vi "Configure Trigger Source [TRG].vi"(8 "error in (no error)":errorcluster, 9 "trigger source (External)":i32(ring)=1 items=["Internal"=3, "External"=1, "Software Trigger Function"=2, "PXI TRIG0 or VXI TTL0"=111, "PXI TRIG1 or VXI TTL1"=112, "PXI TRIG2 or VXI TTL2"=113, "PXI TRIG3 or VXI TTL3"=114, "PXI TRIG4 or VXI TTL4"=115, "PXI TRIG5 or VXI TTL5"=116, "PXI TRIG6 or VXI TTL6"=117, "PXI TRIG7 or VXI TTL7"=118, "ECL0"=119, "ECL1"=120, "PXI Star"=131, "RTSI 0"=141, "RTSI 1"=142, "RTSI 2"=143, "RTSI 3"=144, "RTSI 4"=145, "RTSI 5"=146, "RTSI 6"=147], 10 "channel name (\"CHANNEL1\")":string="CHANNEL1", 11 "CS++Fgen in":refnum<class "CS++Fgen.lvclass">) -> (0 "error out":errorcluster, 3 "CS++Fgen out":refnum<class "CS++Fgen.lvclass">)   [LabVIEW 2013, in "CS++Fgen.lvlib" / "CS++Fgen.lvclass"]
doc: "This VI configures the trigger source for a channel.\n\nNotes:\n\n(1) This VI is part of the IviFgenTrigger [TRG] extension group."
uses:
  CS++Fgen.lvclass
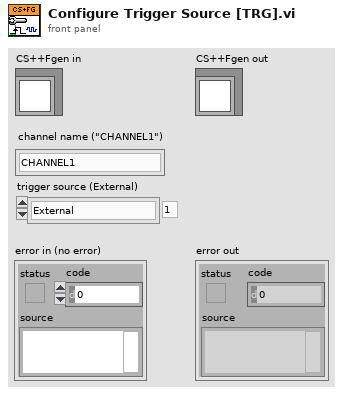
[diagram p1: front panel]
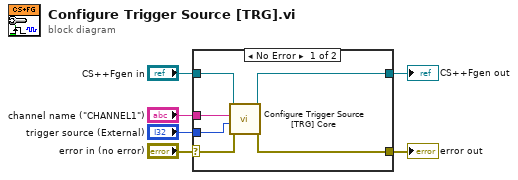
[diagram p0: block diagram]
diagram:
  n1 = case shown="No Error" "error in (no error)" {
    selector: "error in (no error)" -> [w10 w14]
    tunnel: [w9 w14] -> w5
    tunnel: [w11 w13] -> w3
    tunnel: "CS++Fgen in" -> [w12 w13]
    tunnel: "channel name (\"CHANNEL1\")" -> [w8 _]
    tunnel: "trigger source (External)" -> [w7 _]
    frame No Error {
      n2 = call-dynamic "Configure Trigger Source [TRG] Core.vi"("error in (no error)"=w10, "trigger source (External)"=w7, "channel name (\"CHANNEL1\")"=w8, "CS++Fgen in"=w12) -> ("error out"=w9:errorcluster, "CS++Fgen out"=w11:refnum<class "CS++Fgen.lvclass">)  [unwired: 6 in]
    }
    frame Error {
    }
  }
  "error out" <- w5
  "CS++Fgen out" <- w3
